vi "Read Attributes.vi"(11 "Endpoint Connected Msg in":refnum<class "Endpoint Connected Msg.lvclass">) -> (2 "Endpoint":refnum<class "Message Enqueuer.lvclass">)   [LabVIEW 2020, in "Nested Endpoint Caller.lvlib" / "Endpoint Connected Msg.lvclass"]
uses:
  Endpoint Connected Msg.lvclass
  <vilib>/ActorFramework/Message Enqueuer/Message Enqueuer.lvclass
  Endpoint Connected Msg.lvclass/Endpoint Connected Msg.ctl
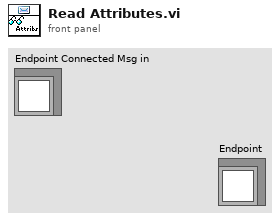
[diagram p1: front panel]
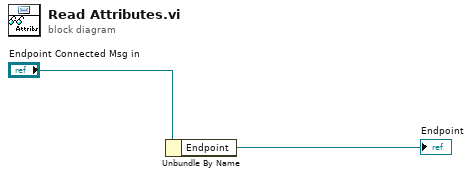
[diagram p0: block diagram]
diagram:
  n1 = Unbundle By Name("Endpoint Connected Msg in") -> ("Endpoint"=→"Endpoint":refnum<class "Message Enqueuer.lvclass">)
